vi "RUSHShoot.vi"(1 "In Cluster":T2) -> (0 "Out Cluster":T1)   [LabVIEW 2012]
panel:
  in  "Highest POT pos":dbl=5.0
  in  "Lowest POT pos":dbl
  in  "ShootPOTToPowConst":dbl=0.2
  in  "Vision Speed Const":dbl=0.75
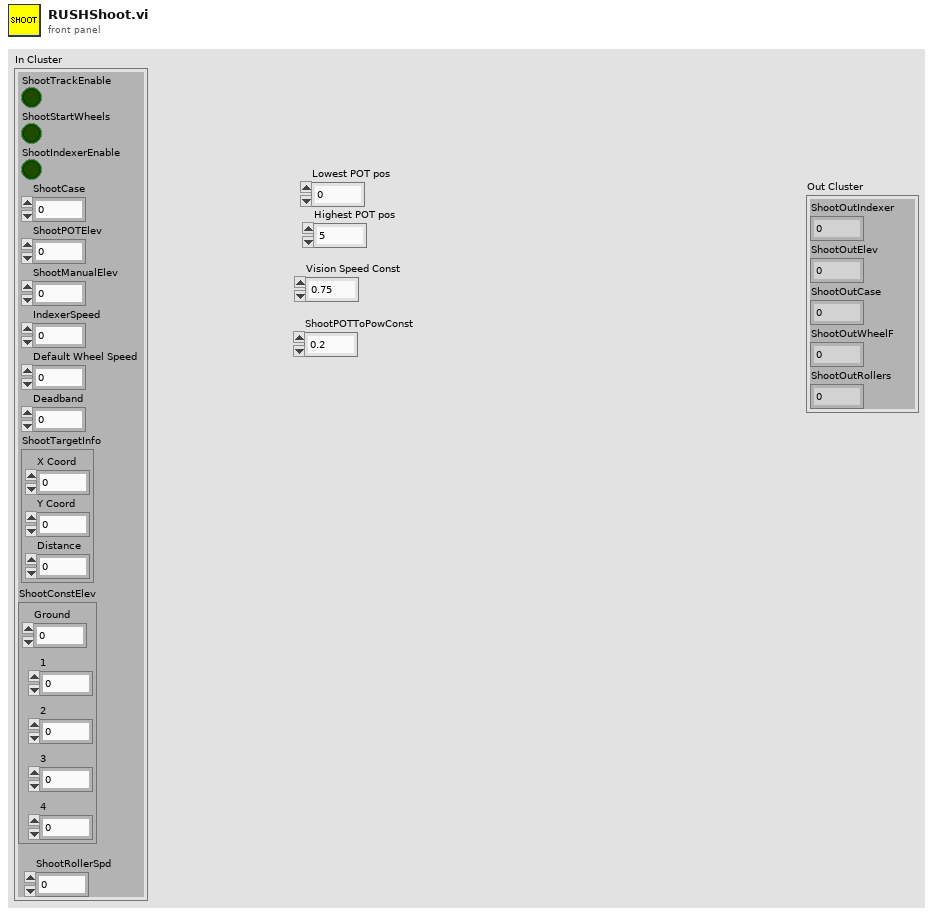
[diagram p1: front panel]
types:
  T1 = cluster{"ShootOutIndexer":dbl, "ShootOutElev":dbl, "ShootOutCase":dbl, "ShootOutWheelF":dbl, "ShootOutRollers":dbl}
  T2 = cluster{"ShootTrackEnable":bool, "ShootStartWheels":bool, "ShootIndexerEnable":bool, "ShootCase":dbl, "ShootPOTElev":dbl, "ShootManualElev":dbl, "IndexerSpeed":dbl, "Default Wheel Speed":dbl, "Deadband":dbl, "ShootTargetInfo":cluster{"X Coord":dbl, "Y Coord":dbl, "Distance":dbl}, "ShootConstElev":cluster{"1":dbl, "2":dbl, "3":dbl, "4":dbl, "Ground":dbl}, "ShootRollerSpd":dbl}
  T3 = cluster{"X Coord":dbl, "Y Coord":dbl, "Distance":dbl}
  T4 = cluster{"1":dbl, "2":dbl, "3":dbl, "4":dbl, "Ground":dbl}
  T5 = cluster{"f":dbl, "y":dbl, "f":dbl, "f":dbl, "f":dbl}
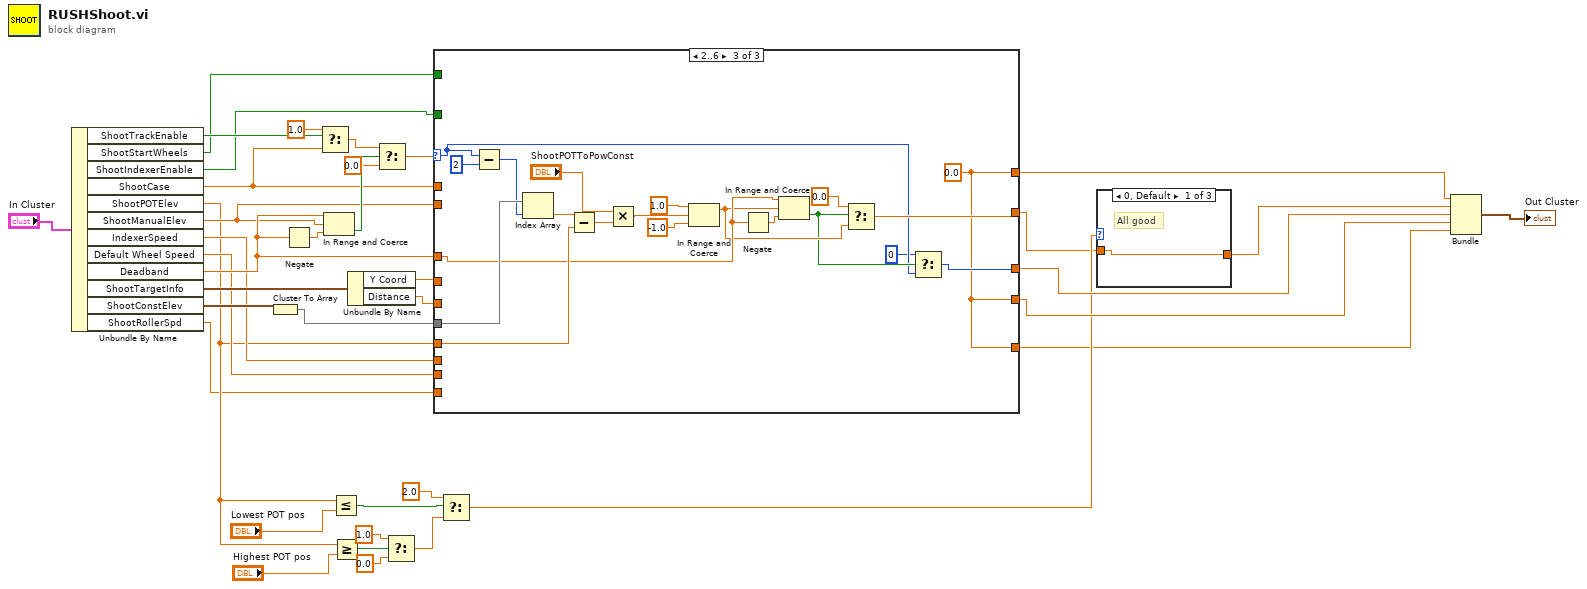
[diagram p0: block diagram]
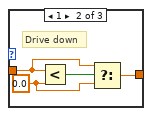
[diagram p2: hidden frame]
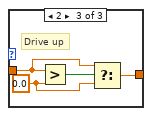
[diagram p3: hidden frame]
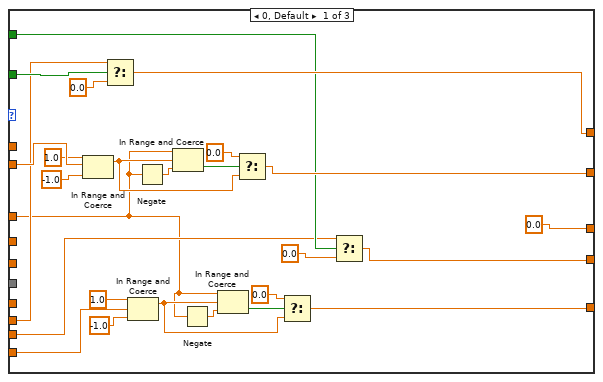
[diagram p4: hidden frame]
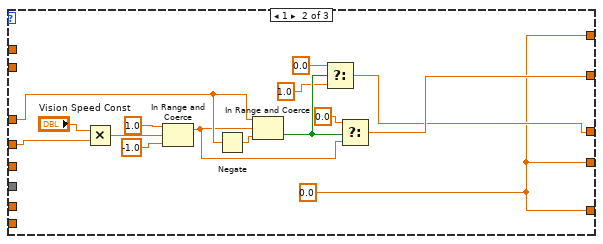
[diagram p5: hidden frame]
diagram:
  n1 = Unbundle By Name("In Cluster") -> ("ShootTrackEnable"=w37:bool, "ShootStartWheels"=w25:bool, "ShootIndexerEnable"=w24:bool, "ShootCase"=w26:dbl, "ShootPOTElev"=w13:dbl, "ShootManualElev"=w23:dbl, "IndexerSpeed"=w16:dbl, "Default Wheel Speed"=w15:dbl, "Deadband"=w27:dbl, "ShootTargetInfo"=w30:T3, "ShootConstElev"=w22:T4, "ShootRollerSpd"=w2:dbl)
  n2 = Cluster To Array(cluster=w22) -> (array=w21:dbl[])
  n3 = Negate(x=w27) -> (-x=w34:dbl)
  n4 = Select(t=1.0, s=w37, f=w26) -> (s? t:f=w35:dbl)
  n5 = In Range and Coerce(upper limit=w27, x=w23, lower limit=w34) -> (In Range?=w33:bool)  [unwired: 1 out]
  n6 = Less Or Equal?(x=w13, y="Lowest POT pos") -> (x <= y?=w7:bool)
  n7 = Greater Or Equal?(x=w13, y="Highest POT pos") -> (x >= y?=w11:bool)
  n8 = Unbundle By Name(w30) -> ("Y Coord"=w29:dbl, "Distance"=w28:dbl)
  n9 = Select(t=w35, s=w33, f=0.0) -> (s? t:f=w31:dbl)
  n10 = Select(t=1.0, s=w11, f=0.0) -> (s? t:f=w8:dbl)
  n11 = case shown="2..6" w31 {
    selector: w31 -> [_ _ w83]
    tunnel: w29 -> [_ w78 _]
    tunnel: w28 -> [_ _ _]
    tunnel: w27 -> [w40 w73 w88]
    tunnel: [0.0 ("upper limit") w67 w81] -> w19
    tunnel: w26 -> [_ _ _]
    tunnel: [w55 w68 w85] -> w4
    tunnel: [w52 w65 w80] -> w18
    tunnel: [w62 w65 w80] -> w20
    tunnel: w25 -> [w53 _ _]
    tunnel: w24 -> [w64 _ _]
    tunnel: w23 -> [w59 _ _]
    tunnel: w21 -> [_ _ w98]
    tunnel: w13 -> [_ _ w95]
    tunnel: w16 -> [w48 _ _]
    tunnel: w15 -> [w49 _ _]
    tunnel: w2 -> [w41 _ _]
    tunnel: [w39 w65 w80] -> w1
    frame 0, Default {
      n12 = In Range and Coerce(upper limit=1.0, x=w59, lower limit=-1.0 ("upper limit")) -> (coerced(x)=w56:dbl)  [unwired: 1 out]
      n13 = Select(t=w48, s=w64, f=0.0) -> (s? t:f=w62:dbl)
      n14 = In Range and Coerce(upper limit=1.0, x=w41, lower limit=-1.0 ("upper limit")) -> (coerced(x)=w46:dbl)  [unwired: 1 out]
      n15 = Negate(x=w40) -> (-x=w60:dbl)
      n16 = In Range and Coerce(upper limit=w40, x=w56, lower limit=w60) -> (In Range?=w58:bool)  [unwired: 1 out]
      n17 = Negate(x=w40) -> (-x=w43:dbl)
      n18 = In Range and Coerce(upper limit=w40, x=w46, lower limit=w43) -> (In Range?=w44:bool)  [unwired: 1 out]
      n19 = Select(t=0.0, s=w58, f=w56) -> (s? t:f=w55:dbl)
      n20 = Select(t=0.0, s=w44, f=w46) -> (s? t:f=w39:dbl)
      n21 = Select(t=w49, s=w53, f=0.0 ("t")) -> (s? t:f=w52:dbl)
    }
    frame 1 {
      w65 = 0.0
      n22 = Multiply(x="Vision Speed Const", y=w78) -> (x*y=w77:dbl)
      n23 = In Range and Coerce(upper limit=1.0, x=w77, lower limit=-1.0 ("upper limit")) -> (coerced(x)=w71:dbl)  [unwired: 1 out]
      n24 = Negate(x=w73) -> (-x=w74:dbl)
      n25 = In Range and Coerce(upper limit=w73, x=w71, lower limit=w74) -> (In Range?=w70:bool)  [unwired: 1 out]
      n26 = Select(t=0.0, s=w70, f=1.0) -> (s? t:f=w67:dbl)
      n27 = Select(t=0.0, s=w70, f=w71) -> (s? t:f=w68:dbl)
    }
    frame 2..6 {
      w80 = 0.0 ("f")
      n28 = Subtract(x=w83, y=2) -> (x-y=w97:i32)
      n29 = Index Array(array=w98, index=w97) -> (element=w96:dbl)
      n30 = Subtract(x=w96, y=w95) -> (x-y=w94:dbl)
      n31 = Multiply(x="ShootPOTToPowConst", y=w94) -> (x*y=w89:dbl)
      n32 = In Range and Coerce(upper limit=1.0, x=w89, lower limit=-1.0 ("upper limit")) -> (coerced(x)=w86:dbl)  [unwired: 1 out]
      n33 = Negate(x=w88) -> (-x=w90:dbl)
      n34 = In Range and Coerce(upper limit=w88, x=w86, lower limit=w90) -> (In Range?=w84:bool)  [unwired: 1 out]
      n35 = Select(t=0.0, s=w84, f=w86) -> (s? t:f=w85:dbl)
      n36 = Select(t=0, s=w84, f=w83) -> (s? t:f=w81:i32)
    }
  }
  n37 = Select(t=2.0, s=w7, f=w8) -> (s? t:f=w5:dbl)
  n38 = case shown="0, Default" w5 {
    tunnel: w4 -> [w100 w102 w106]
    tunnel: [w100 w101 w105] -> w3
    frame 0, Default {
      # "All good"
    }
    frame 1 {
      w103 = 0.0 ("y")
      # "Drive down"
      n39 = Less?(x=w102, y=w103) -> (x < y?=w104:bool)
      n40 = Select(t=w102, s=w104, f=w103) -> (s? t:f=w101:dbl)
    }
    frame 2 {
      w107 = 0.0 ("y")
      # "Drive up"
      n41 = Greater?(x=w106, y=w107) -> (0:w108:bool)
      n42 = Select(t=w106, s=w108, f=w107) -> (s? t:f=w105:dbl)
    }
  }
  n43 = Bundle("f"=w20, "y"=w3, "f"=w19, "f"=w18, "f"=w1) -> (→"Out Cluster":T5)  [unwired: 1 in]
